vi "Servo-Centerization.vi"(1 "Camera Angle":dbl=23.5, 2 "Cartez":dbl) -> (0 "Rounded Error":dbl)   [LabVIEW 2011]
panel:
  out "Error":dbl
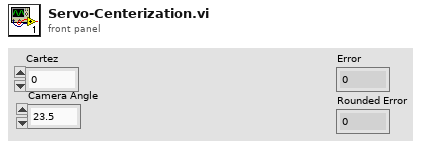
[diagram p1: front panel]
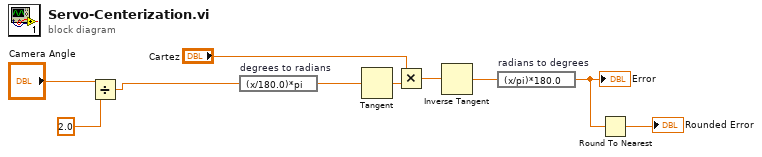
[diagram p0: block diagram]
diagram:
  n1 = Divide(x="Camera Angle", y=2.0) -> (x/y=w1:dbl)
  n2 = expression code="(x/180.0)*pi" "degrees to radians"(w1) -> (w6:dbl)
  n3 = Tangent(1:w6) -> (0:w10:dbl)
  n4 = Multiply(x="Cartez", y=w10) -> (x*y=w7:dbl)
  n5 = Inverse Tangent(1:w7) -> (0:w8:dbl)
  n6 = expression code="(x/pi)*180.0" "radians to degrees"(w8) -> (w4:dbl)
  "Error" <- w4
  n7 = Round To Nearest(number=w4) -> (nearest integer value=→"Rounded Error":dbl)
